vi "CurenessTesting.vi"() -> ()   [LabVIEW 2017]
uses:
  Shared Components/Config Manager Class/Type Definitions/Potting Parameters.ctl
  <vilib>/Utility/error.llb/DialogType.ctl
  Shared Components/Config Manager Class/Type Definitions/Camera Enum.ctl
  Shared Components/Gantry Class/Type Definitions/Init_Modes.ctl
  Shared Components/Gantry Class/Type Definitions/Virtual Modes.ctl
  Shared Components/Config Manager Class/Type Definitions/Potting Surface Type.ctl
  Shared Components/Gantry Class/Gantry Class.lvclass
  Shared Components/SyringeTool Class/SyringeTool Class.lvclass
  Shared Components/WorkTable Class/WorkTable Class.lvclass
  Shared Components/Vec3d Class/Vec3d Class.lvclass
panel:
  out "error out":errorcluster
  in  "Potting Parameters":T1={"Curing Param A"=0.0, "Curing Param B"=0.0, "Speed Nominal"=0.5, "Time Nominal"=2.0, "Turn-on Time"=0.5, "Turn-off Time"=0.1, "Safe Height Offset"=0.0, "Tip Height"=0.18, "Width of Line"=0.0, "Number of lines"=1.0, "Distance between lines"=0.1}
  out "Image":T2(plugin-control)
  in  "stop":bool
  in  "Config Folder":path=path "C:/Users/Husker/Desktop/gantry/Config"
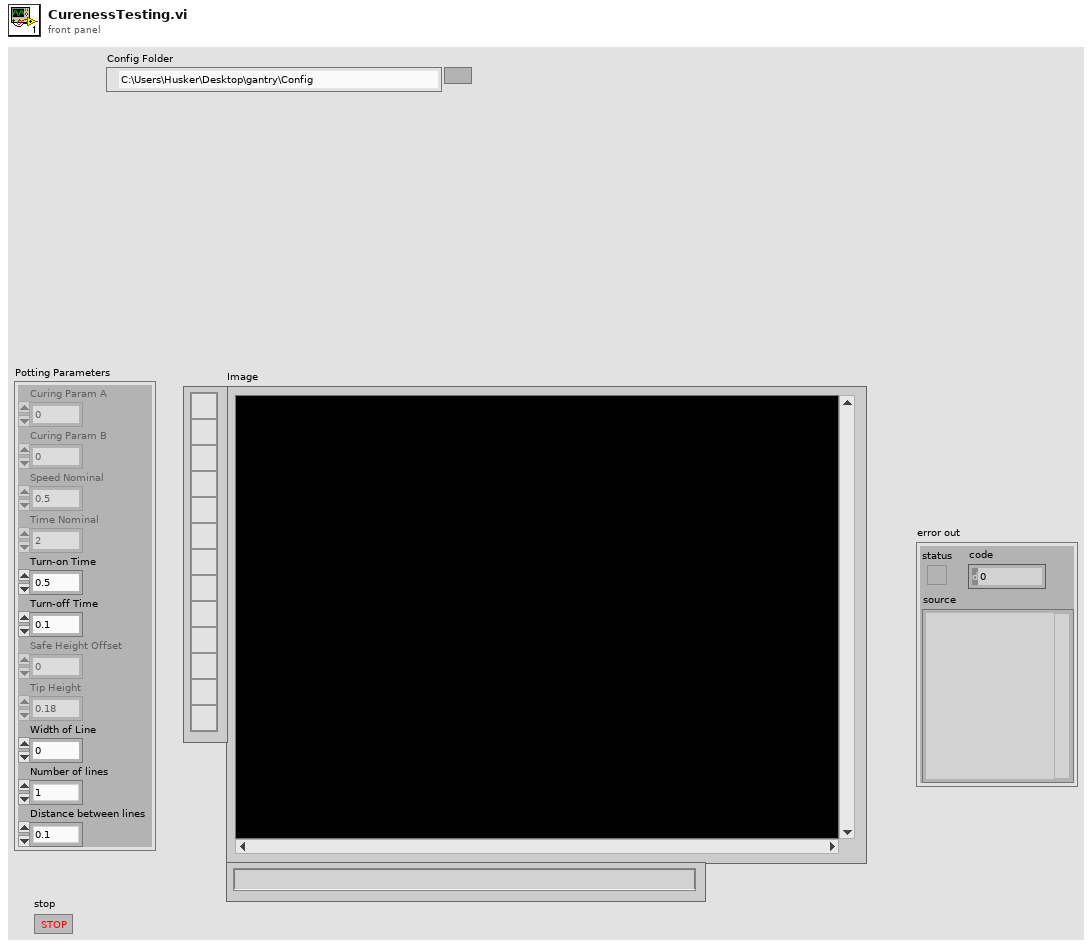
[diagram p1: front panel]
types:
  T1 = typedef "Potting Parameters.ctl" = cluster{"Curing Param A":dbl, "Curing Param B":dbl, "Speed Nominal":dbl, "Time Nominal":dbl, "Turn-on Time":dbl, "Turn-off Time":dbl, "Safe Height Offset":dbl, "Tip Height":dbl, "Width of Line":dbl, "Number of lines":dbl, "Distance between lines":dbl}
  T2 = typedef "IMAQ Image.ctl" = refnum<image>
  T3 = typedef "Virtual Modes.ctl" = enum16{"Nonvirtual", "Pseudovirtual", "Virtual"}
  T4 = typedef "Init_Modes.ctl" = enum16{"Full", "Robot Only", "Dispenser Only", "Cameras Only", "Robot and Cameras", "Robot and Cameras and Dispenser", "Manifold Only"}
  T5 = typedef "Camera Enum.ctl" = enum16{"GANTRY HEAD", "NEEDLE CALIBRATION X", "NEEDLE CALIBRATION Y", "STAND CAMERA", "SIMRAN WEBCAM"}
  T6 = typedef "DialogType.ctl" = u16
  T7 = typedef "Worktable_Syringe.ctl" = cluster{"Syringe Holder":enum16{"Empty", "Populated", "Calibrated"}, "Mixing Time":timestamp, "Tip Offset":refnum<class "Vec3d Class.lvclass">}
  T8 = typedef "Potting Surface Type.ctl" = enum16{"default", "hdi_edge_pads", "bbm_edge_pads", "address_pads"}
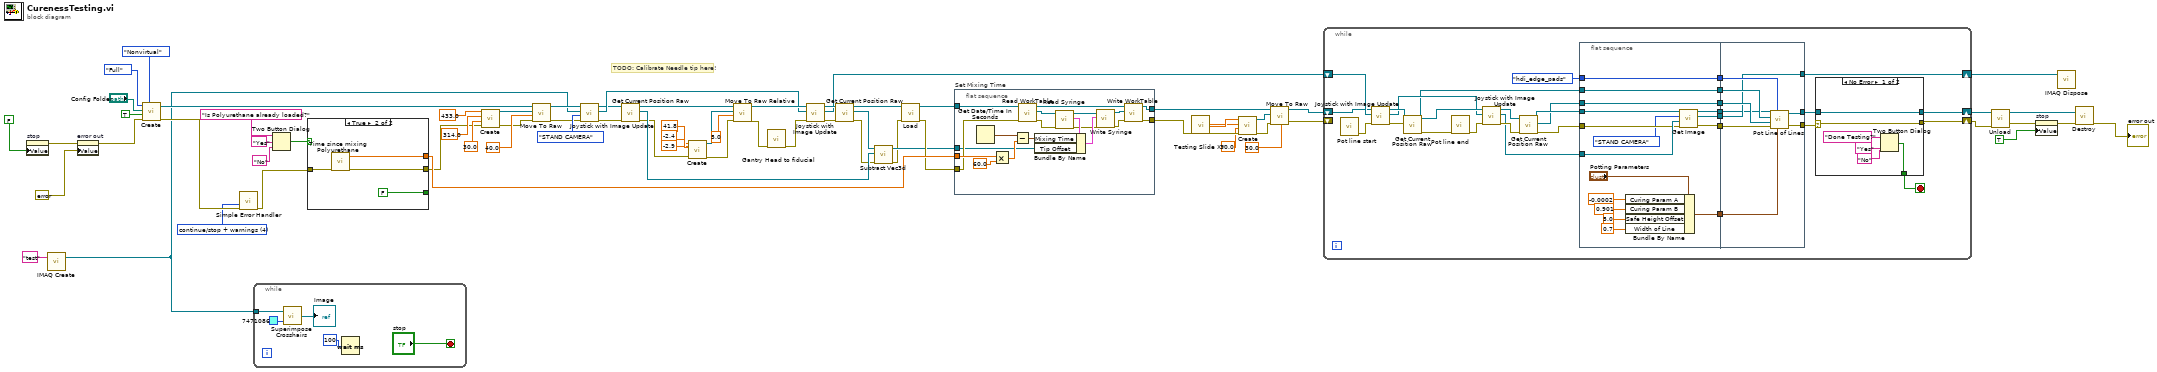
[diagram p0: block diagram]
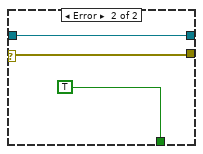
[diagram p2: hidden frame]
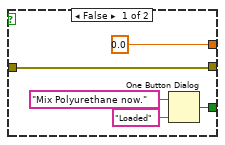
[diagram p3: hidden frame]
diagram:
  w62 = T6 4 items=["no dialog", "OK message", "continue or stop message", "OK message + warnings", "continue/stop + warnings"] ("type of dialog (OK msg:1)")
  # "TODO: Calibrate Needle tip here!"
  n1 = property on="stop" class="Bool (strict)"("Value"=FALSE) -> (error out=w4:errorcluster)  [unwired: 2 in, 1 out]
  n2 = call "IMAQ Create"("Image Name"="test") -> ("New Image"=w31:T2)  [unwired: 4 in, 1 out]
  n3 = property on="error out" class="Clust (strict)"(error in=w4, "Value"=errorcluster {"status"=FALSE, "code"=0, "source"=""} ("error in (no error)")) -> (error out=w1:errorcluster)  [unwired: 1 in, 1 out]
  n4 = call "Create.vi"("Virtual Mode"=Virtual_Modes."Nonvirtual", "error in"=w1, "HOME?"=TRUE, "Config Folder"="Config Folder", "Init Mode"=Init_Modes."Full") -> ("error out"=w64:errorcluster, "Gantry out"=w55:refnum<class "Gantry Class.lvclass">)  [unwired: 5 in]
  n5 = call <vilib>:"Simple Error Handler.vi"("type of dialog (OK msg:1)"=w62, "error in (no error)"=w64) -> ("error out"=w63:errorcluster)  [unwired: 3 in, 4 out]
  n6 = while {
    tunnel: w31 -> [w76]
    stop <- "stop" stop-if-true
    n7 = call "Superimpose Crosshairs.vi"("Grid Line Color"=u32 7471086, "Refnum in"=w76) -> ("Refnum out"=→"Image":T2)
    n8 = Wait (ms)(milliseconds to wait=u32 100) -> ()  [unwired: 1 out]
  }
  n9 = Two Button Dialog(message="Is Polyurethane already loaded?", 1:"No" ("F button name (\"Cancel\")"), 2:"Yes" ("T button name (\"OK\")")) -> (T button?=w68:bool)
  n10 = case shown="True" w68 {
    tunnel: w63 -> [w79 w86]
    tunnel: [w79 w85] -> w54
    tunnel: [0.0 ("minutes") w87] -> w72
    tunnel: [w80 FALSE ("true")] -> _
    frame False {
      n11 = One Button Dialog(message="Mix Polyurethane now.", button name ("OK")="Loaded") -> (true=w80:bool)
    }
    frame True {
      n12 = call "Time since mixing Polyurethane"("error in (no error)"=w86) -> ("minutes"=w87:dbl, "error out"=w85:errorcluster)  [unwired: 16 in, 1 out]
    }
  }
  n13 = call "Create.vi"("error in"=w54, "Z"=30.0, "Y"=314.0, "X"=433.0) -> ("error out"=w59:errorcluster, "Vec3d Class out"=w61:refnum<class "Vec3d Class.lvclass">)  [unwired: 6 in]
  n14 = call-dynamic "Move To Raw.vi"("error in"=w59, "Speed"=40.0, "Destination"=w61, "Gantry in"=w55) -> ("error out"=w33:errorcluster, "Gantry out"=w34:refnum<class "Gantry Class.lvclass">)  [unwired: 6 in]
  n15 = call-dynamic "Joystick with Image Update.vi"("error in (no error)"=w33, "Camera Name"=Camera_Enum."STAND CAMERA", "Image In"=w31, "Gantry Class in"=w34) -> ("error out"=w39:errorcluster, "Image Out"=w42:T2, "Gantry Class out"=w40:refnum<class "Gantry Class.lvclass">)  [unwired: 5 in]
  n16 = call-dynamic "Get Current Position Raw.vi"("error in"=w39, "Gantry in"=w40) -> ("error out"=w36:errorcluster, "Vec3d Class out"=w37:refnum<class "Vec3d Class.lvclass">, "Gantry out"=w38:refnum<class "Gantry Class.lvclass">)  [unwired: 7 in]
  n17 = call "Create.vi"("error in"=w36, "Z"=-2.9, "Y"=-2.4, "X"=41.8) -> ("error out"=w41:errorcluster, "Vec3d Class out"=w46:refnum<class "Vec3d Class.lvclass">)  [unwired: 6 in]
  n18 = call-dynamic "Move To Raw Relative.vi"("error in"=w41, "Speed(mm/s)"=5.0 ("Speed"), "Delta"=w46, "Gantry in"=w38) -> ("error out"=w43:errorcluster, "Gantry out"=w44:refnum<class "Gantry Class.lvclass">)  [unwired: 6 in]
  n19 = call "Gantry Head to fiducial"("error in (no error)"=w43) -> ("error out"=w50:errorcluster)  [unwired: 9 in, 1 out]
  n20 = call-dynamic "Joystick with Image Update.vi"("error in (no error)"=w50, "Image In"=w42, "Gantry Class in"=w44) -> ("error out"=w52:errorcluster, "Image Out"=w21:T2, "Gantry Class out"=w53:refnum<class "Gantry Class.lvclass">)  [unwired: 6 in]
  n21 = call-dynamic "Get Current Position Raw.vi"("error in"=w52, "Gantry in"=w53) -> ("error out"=w28:errorcluster, "Vec3d Class out"=w51:refnum<class "Vec3d Class.lvclass">, "Gantry out"=w30:refnum<class "Gantry Class.lvclass">)  [unwired: 7 in]
  n22 = call "Subtract Vec3d.vi"("error in (no error)"=w28, "Vec3d in 2"=w37, "Vec3d in 1"=w51) -> ("error out"=w27:errorcluster, "Vec3d Class out"=w29:refnum<class "Vec3d Class.lvclass">)  [unwired: 7 in]
  n23 = call "Load.vi"("error in"=w27, "Gantry in"=w30) -> ("error out"=w66:errorcluster, "SyringeTool out"=w67:refnum<class "SyringeTool Class.lvclass">)  [unwired: 8 in]
  n24 = flat-sequence "Set Mixing Time" {
    tunnel: w67 -> [w102]
    tunnel: w72 -> [w106]
    tunnel: w66 -> [w101]
    tunnel: [w90] -> w23
    tunnel: [w89] -> w24
    tunnel: w29 -> [w88]
    frame #0 {
      n25 = Get Date/Time In Seconds() -> (seconds since 1Jan1904=w104:timestamp)
      n26 = Multiply(x=w106, y=60.0) -> (x*y=w103:dbl)
      n27 = Subtract(x=w104, y=w103) -> (x-y=w98:timestamp)
      n28 = call-dynamic "Read WorkTable.vi"("error in"=w101, "Gantry Class in"=w102) -> ("error out"=w93:errorcluster, "WorkTable Class.lvclass"=w100:refnum<class "WorkTable Class.lvclass">, "Gantry Class out"=w95:refnum<class "SyringeTool Class.lvclass">)  [unwired: 7 in]
      n29 = call "Read Syringe.vi"("error in"=w93, "WorkTable in"=w100) -> ("error out"=w92:errorcluster, "Syringe"=w99:T7, "WorkTable out"=w96:refnum<class "WorkTable Class.lvclass">)  [unwired: 7 in]
      n30 = Bundle By Name(cluster=w99, "Mixing Time"=w98, "Tip Offset"=w88) -> (w97:T7)
      n31 = call-dynamic "Write Syringe.vi"("error in (no error)"=w92, "Syringe"=w97, "WorkTable Class in"=w96) -> ("error out"=w91:errorcluster, "WorkTable Class out"=w94:refnum<class "WorkTable Class.lvclass">)  [unwired: 7 in]
      n32 = call-dynamic "Write WorkTable.vi"("error in (no error)"=w91, "WorkTable Class.lvclass"=w94, "Gantry Class in"=w95) -> ("error out"=w89:errorcluster, "Gantry Class out"=w90:refnum<class "SyringeTool Class.lvclass">)  [unwired: 7 in]
    }
  }
  n33 = call "Testing Slide XY"("error in (no error)"=w24) -> ("Y"=w19:dbl, "X"=w20:dbl, "error out"=w15:errorcluster)  [unwired: 15 in, 1 out]
  n34 = call "Create.vi"("error in"=w15, "Z"=30.0, "Y"=w19, "X"=w20) -> ("error out"=w16:errorcluster, "Vec3d Class out"=w18:refnum<class "Vec3d Class.lvclass">)  [unwired: 6 in]
  n35 = call-dynamic "Move To Raw.vi"("error in"=w16, "Speed"=30.0, "Destination"=w18, "Gantry in"=w23) -> ("error out"=w22:errorcluster, "Gantry out"=w13:refnum<class "SyringeTool Class.lvclass">)  [unwired: 6 in]
  n36 = while {
    shift-right: [w113] -> w25
    shift-left: w21 -> [w131]
    shift-right: [w107] -> w11
    shift-left: w22 -> [_]
    shift-right: [w108] -> w12
    shift-left: w13 -> [w111]
    stop <- w121 stop-if-true
    n37 = call "Pot line start"() -> ("error out"=w124:errorcluster)  [unwired: 10 in, 1 out]
    n38 = call-dynamic "Joystick with Image Update.vi"("error in (no error)"=w124, "Image In"=w131, "Gantry Class in"=w111) -> ("error out"=w125:errorcluster, "Image Out"=w134:T2, "Gantry Class out"=w136:refnum<class "SyringeTool Class.lvclass">)  [unwired: 6 in]
    n39 = call-dynamic "Get Current Position Raw.vi"("error in"=w125, "Gantry in"=w136) -> ("error out"=w123:errorcluster, "Vec3d Class out"=w129:refnum<class "Vec3d Class.lvclass">, "Gantry out"=w135:refnum<class "SyringeTool Class.lvclass">)  [unwired: 7 in]
    n40 = call "Pot line end"("error in (no error)"=w123) -> ("error out"=w122:errorcluster)  [unwired: 9 in, 1 out]
    n41 = call-dynamic "Joystick with Image Update.vi"("error in (no error)"=w122, "Image In"=w134, "Gantry Class in"=w135) -> ("error out"=w132:errorcluster, "Image Out"=w115:T2, "Gantry Class out"=w133:refnum<class "SyringeTool Class.lvclass">)  [unwired: 6 in]
    n42 = call-dynamic "Get Current Position Raw.vi"("error in"=w132, "Gantry in"=w133) -> ("error out"=w126:errorcluster, "Vec3d Class out"=w128:refnum<class "Vec3d Class.lvclass">, "Gantry out"=w130:refnum<class "SyringeTool Class.lvclass">)  [unwired: 7 in]
    n43 = flat-sequence {
      tunnel: w126 -> [w141]
      tunnel: Potting_Surface_Type."hdi_edge_pads" ("Potting Surface Type") -> [w150]
      tunnel: w128 -> [w151]
      tunnel: w129 -> [w152]
      tunnel: w130 -> [w142]
      tunnel: [w152] -> w120
      tunnel: [w151] -> w119
      tunnel: [w150] -> w118
      tunnel: [w140] -> w117
      tunnel: [w148] -> w116
      tunnel: w115 -> [w143]
      tunnel: [w138] -> w114
      tunnel: [w137] -> w112
      tunnel: w120 -> [w161]
      tunnel: w119 -> [w160]
      tunnel: w118 -> [w159]
      tunnel: w117 -> [w158]
      tunnel: w116 -> [w157]
      tunnel: [w156] -> w113
      tunnel: w114 -> [w156]
      tunnel: w112 -> [w155]
      tunnel: [w154] -> w110
      tunnel: [w153] -> w109
      frame #0 {
        n44 = Bundle By Name(cluster="Potting Parameters", "Curing Param A"=-0.0002, "Curing Param B"=0.901, "Safe Height Offset"=5.0, "Width of Line"=0.7 ("Pot Length Scale")) -> (w148:T1)
        n45 = call-dynamic "Get Image.vi"("error in"=w141, "Image In"=w143, "Camera Name"=Camera_Enum."STAND CAMERA", "Gantry in"=w142) -> ("error out"=w140:errorcluster, "Image Out"=w138:T2, "Gantry out"=w137:refnum<class "SyringeTool Class.lvclass">)  [unwired: 4 in, 1 out]
      }
      frame #1 {
        n46 = call "Pot Line of Lines.vi"("Potting Parameters"=w157, "Potting Surface Type"=w159, "error in (no error)"=w158, "End Position"=w160, "Start Position"=w161, "SyringeTool Class in"=w155) -> ("error out"=w153:errorcluster, "SyringeTool Class out"=w154:refnum<class "SyringeTool Class.lvclass">)  [unwired: 4 in]
      }
    }
    n47 = case shown="No Error" w109 {
      selector: w109 -> [w163 w170]
      tunnel: [w163 w170] -> w107
      tunnel: [w164 TRUE ("Done Testing?")] -> w121
      tunnel: w110 -> [w162 w168]
      tunnel: [w162 w168] -> w108
      frame No Error {
        n48 = Two Button Dialog(message="Done Testing?", 1:"No" ("F button name (\"Cancel\")"), 2:"Yes" ("T button name (\"OK\")")) -> (T button?=w164:bool)
      }
      frame Error {
      }
    }
  }
  n49 = call "Unload.vi"("error in"=w11, "SyringeTool in"=w12) -> ("error out"=w6:errorcluster, "Gantry out"=w10:refnum<class "Gantry Class.lvclass">)  [unwired: 8 in]
  n50 = property on="stop" class="Bool (strict)"(error in=w6, "Value"=TRUE ("stop")) -> (error out=w5:errorcluster)  [unwired: 1 in, 1 out]
  n51 = call "IMAQ Dispose"("Image"=w25) -> ()  [unwired: 5 in, 1 out]
  n52 = call "Destroy.vi"("error in"=w5, "Gantry Class in"=w10) -> ("error out"=→"error out":errorcluster)  [unwired: 9 in]
